vi "LABVIEW上位机 - 报警灯.vi"() -> ()   [LabVIEW 2017]
uses:
  <vilib>/Instr/_visa.llb/VISA Configure Serial Port (Instr).vi
panel:
  out "Chart4":u8(graph)
  out "Chart3":u8(graph)
  out "Chart 1":u8(graph)
  out "Chart2":u8(graph)
  out "报警灯4":bool
  out "报警灯3":bool
  in  "ãÐÖµ4":dbl
  out "4号（°C）":dbl
  in  "ãÐÖµ3":dbl
  out "3号（°C）":dbl
  in  "ãÐÖµ2":dbl
  out "报警灯2":bool
  in  "ãÐÖµ1":dbl
  out "报警灯1":bool
  out "2号（°C）":dbl
  in  "stop":bool
  in  "串口号":refnum<visa-resource-name>
  out "1号（°C）":dbl
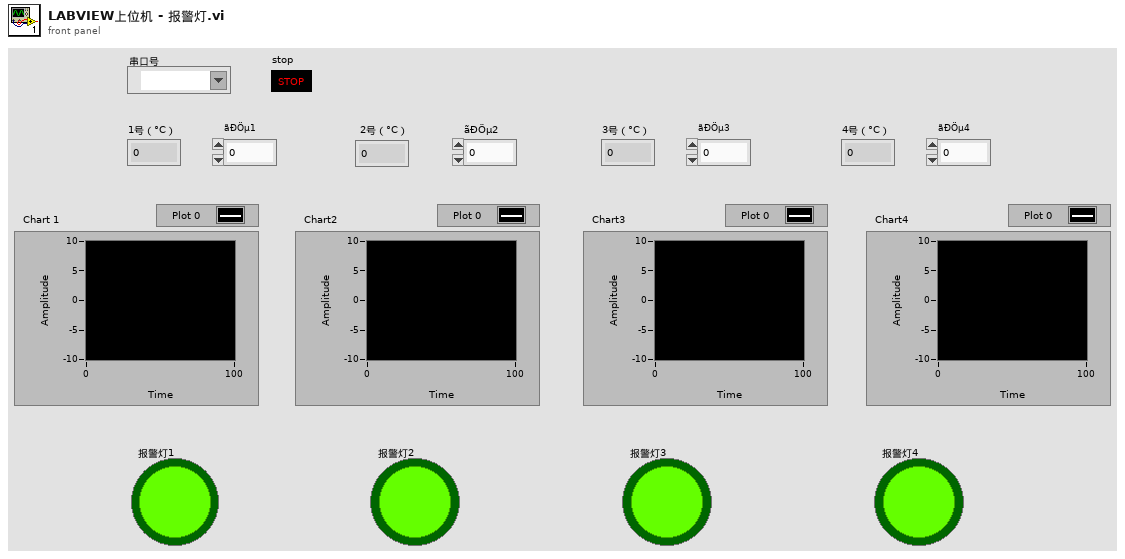
[diagram p1: front panel]
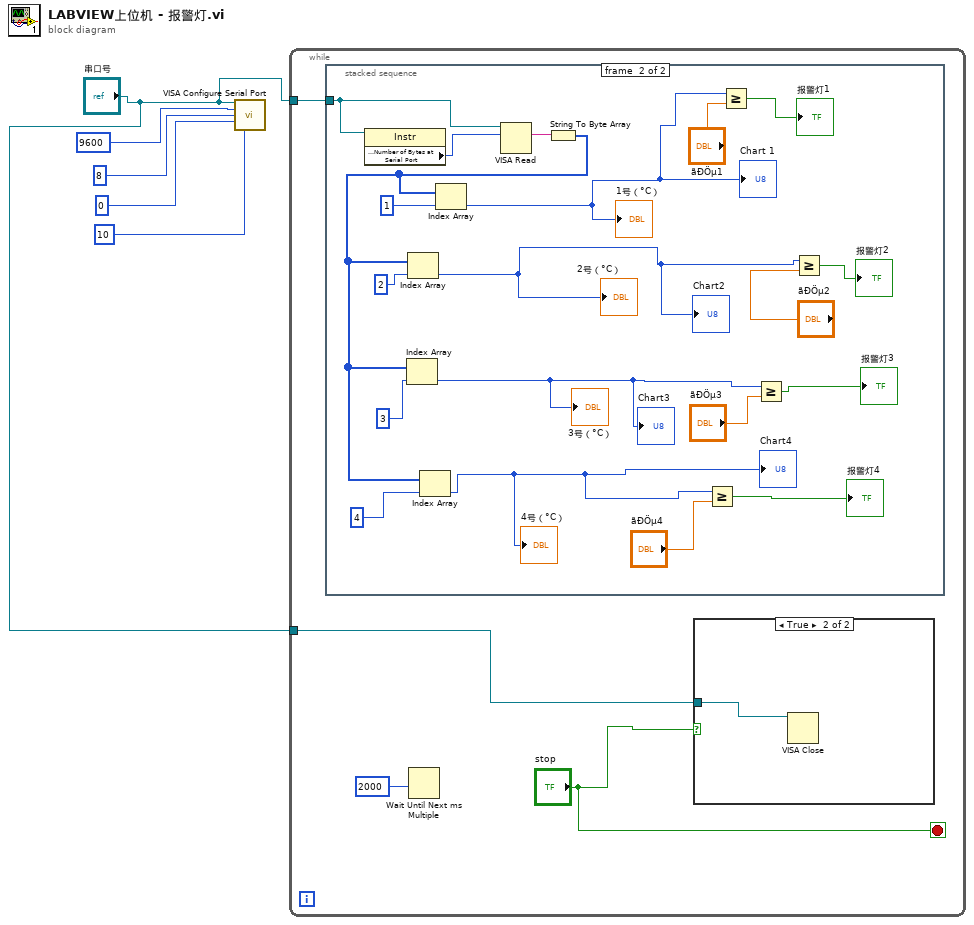
[diagram p0: block diagram]
diagram:
  n1 = call-poly "VISA Configure Serial Port"("VISA resource name"="串口号", "baud rate (9600)"=9600, "data bits (8)"=8, "parity (0:none)"=0, "stop bits (10: 1 bit)"=10) -> ()  [unwired: 9 in, 2 out]
  n2 = while {
    tunnel: "串口号" -> [w9]
    tunnel: "串口号" -> [w8]
    stop <- "stop" stop-if-true
    n3 = stacked-sequence {
      tunnel: w9 -> [_ w28]
      frame #0 {
      }
      frame #1 {
        n4 = property class="Instr"(reference=w28) -> ("Serial Settings:Number of Bytes at Serial Port"=w27:u32)  [unwired: 1 in, 2 out]
        n5 = VISA Read(VISA resource name=w28, byte count=w27) -> (read buffer=w26:string)  [unwired: 1 in, 3 out]
        n6 = String To Byte Array(string=w26) -> (unsigned byte array=w19:u8[])
        n7 = Index Array(array=w19, index=3) -> (element=w12:u8)
        "3号（°C）" <- w12
        "Chart3" <- w12
        n8 = Index Array(array=w19, index=2) -> (element=w13:u8)
        "2号（°C）" <- w13
        "Chart2" <- w13
        n9 = Index Array(array=w19, index=4) -> (element=w11:u8)
        "4号（°C）" <- w11
        "Chart4" <- w11
        n10 = Index Array(array=w19, index=1) -> (element=w14:u8)
        "1号（°C）" <- w14
        "Chart 1" <- w14
        n11 = Greater Or Equal?(x=w11, y="ãÐÖµ4") -> (x >= y?=→"报警灯4":bool)
        n12 = Greater Or Equal?(x=w14, y="ãÐÖµ1") -> (x >= y?=→"报警灯1":bool)
        n13 = Greater Or Equal?(x=w12, y="ãÐÖµ3") -> (x >= y?=→"报警灯3":bool)
        n14 = Greater Or Equal?(x=w13, y="ãÐÖµ2") -> (x >= y?=→"报警灯2":bool)
      }
    }
    n15 = Wait Until Next ms Multiple(millisecond multiple=2000) -> ()  [unwired: 1 out]
    n16 = case shown="True" "stop" {
      tunnel: w8 -> [_ w10]
      frame False {
      }
      frame True {
        n17 = VISA Close(VISA resource name=w10) -> ()  [unwired: 1 in, 1 out]
      }
    }
  }
